vi "Interface.vi"() -> ()   [LabVIEW 2019, in "Command Interface.lvclass"]
uses:
  Command Interface.lvclass
  Robot/Universal Robot/Universal Robot.lvclass
  C:/_Code/Development/Sub-Zero Functional Test/standard hardware/Universal Robots/UR LabVIEW Interface/Classes/Application/Application Interfaces/Application Interface/Application Interface.lvclass
  Application.lvclass
  Application Interface/Application Interface.lvclass
panel:
  in  "Command":u16(ring) items=["Load", "Play", "Stop", "Pause", "Quit", "Shutdown", "Running", "Robotmode", "get loaded program", "popup", "close popup", "addToLog", "IsProgramSaved", "programState", "PolyscopeVersion", "set operational mode", "clear operational mode", "power on", "power off", "brake release", "safetystatus", "unlock protective stop", "close safety popup", "load installation", "restart safety", "get operational mode", "is in remote control", "get serial number", "get robot model", "generate flight report", "generate support file"]
  in  "Input":string
  out "Input Type":string
  in  "send":bool
  out "Return Status":string
  out "Data":string
  out "warning":string
  in  "interface":refnum<class "Command Interface.lvclass">
  in  "robot":refnum<class "Universal Robot.lvclass">
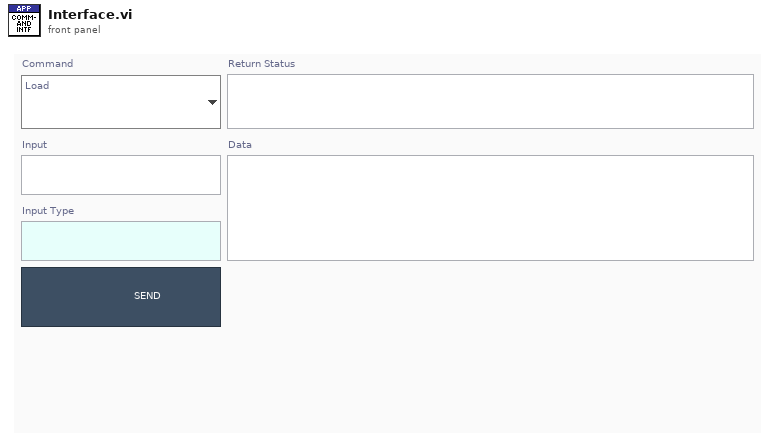
[diagram p1: front panel]
types:
  T1 = enum8{"Enabled", "Disabled", "Disabled and Grayed Out"}
  T2 = typedef "Application.lvclass/FrontPanelControls.ctl" = cluster{"Operation Interface":refnum<vi>, "Program Interface":refnum<vi>, "Command Interface":refnum<vi>, "Socket Interface":refnum<vi>, "Error Interface":refnum<vi>}
  T3 = typedef "Universal Robot.lvclass/PolyScopeCommand.ctl" = cluster{"Command":string, "Input":bool, "Input Type":string, "Remote Mode Required":bool, "Min Version":T4, "Deprecated":bool}
  T4 = typedef "Universal Robot.lvclass/PolyScopeVersion.ctl" = cluster{"Major":i32, "Minor":i32, "Fix":i32, "Build":i32}
  T5 = typedef "Universal Robot.lvclass/RobotStatus.ctl" = cluster{"Robot Mode":T6, "Operational Mode":T7, "Safety Status":T8, "Remote Control":bool}
  T6 = typedef "Universal Robot.lvclass/RobotMode.ctl" = enum16{"INVALID", "NO_CONTROLLER", "DISCONNECTED", "CONFIRM_SAFETY", "BOOTING", "POWER_OFF", "POWER_ON", "IDLE", "BACKDRIVE", "RUNNING"}
  T7 = typedef "Universal Robot.lvclass/OperationalMode.ctl" = enum16{"NONE", "MANUAL", "AUTOMATIC"}
  T8 = typedef "Universal Robot.lvclass/SafetyStatus.ctl" = enum16{"INVALID", "NORMAL", "REDUCED", "PROTECTIVE_STOP", "RECOVERY", "SAFEGUARD_STOP", "SYSTEM_EMERGENCY_STOP", "ROBOT_EMERGENCY_STOP", "VIOLATION", "FAULT", "AUTOMATIC_MODE_SAFEGAURD_STOP", "SYSTEM_THREE_POSITION_ENABLING_STOP"}
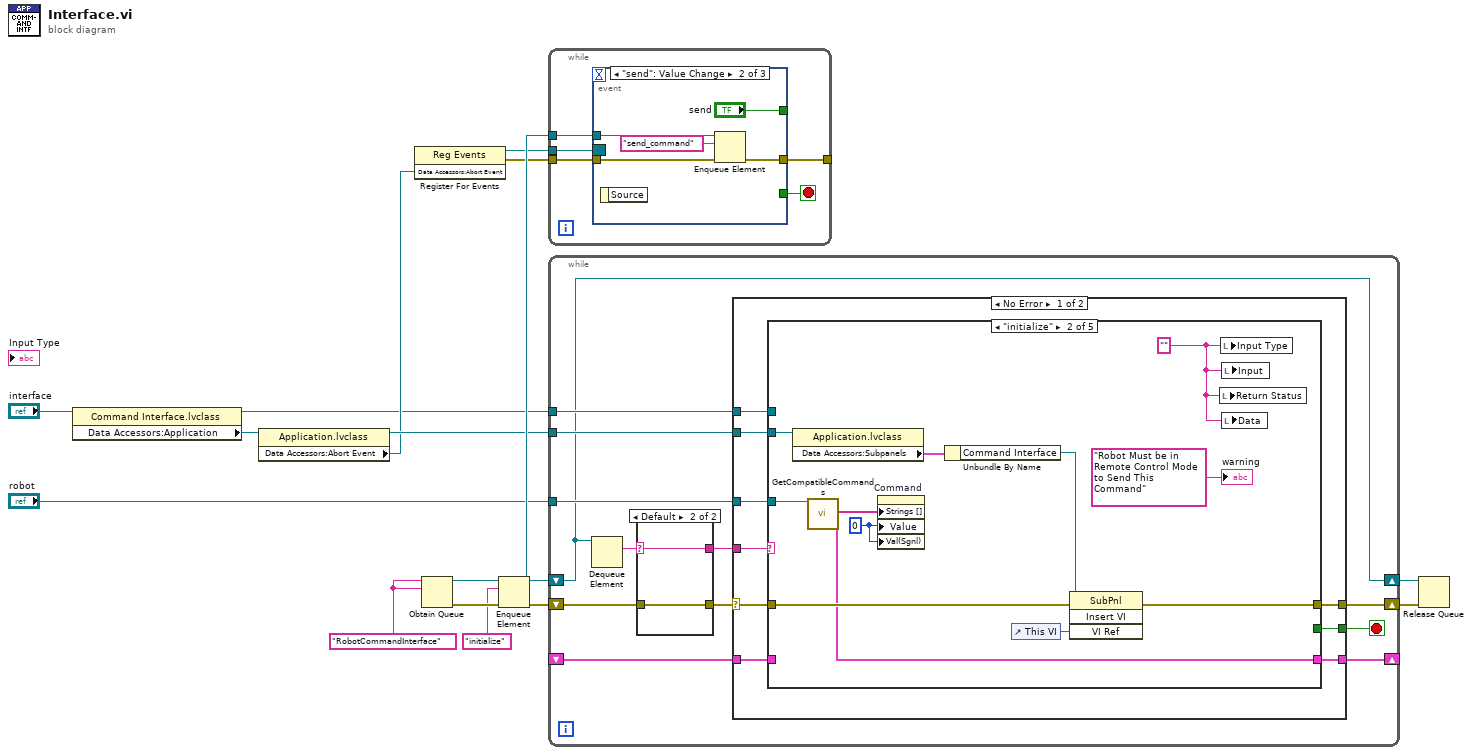
[diagram p0: block diagram]
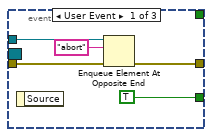
[diagram p2: hidden frame]
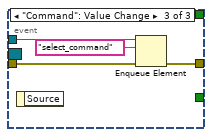
[diagram p3: hidden frame]
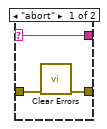
[diagram p4: hidden frame]
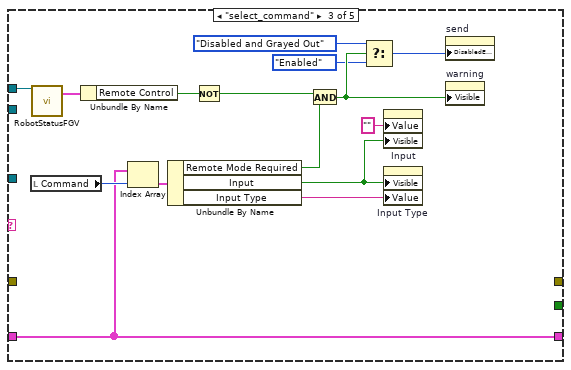
[diagram p6: hidden frame]
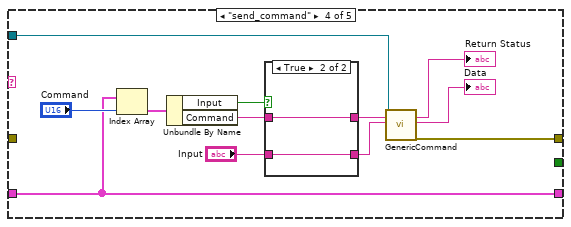
[diagram p7: hidden frame]
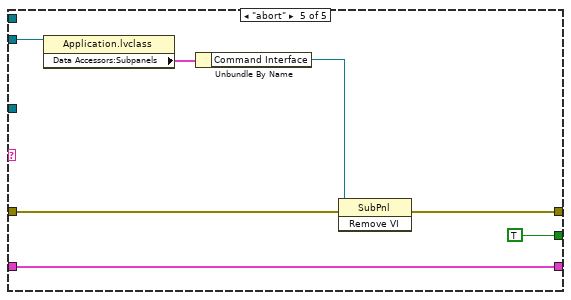
[diagram p9: hidden frame]
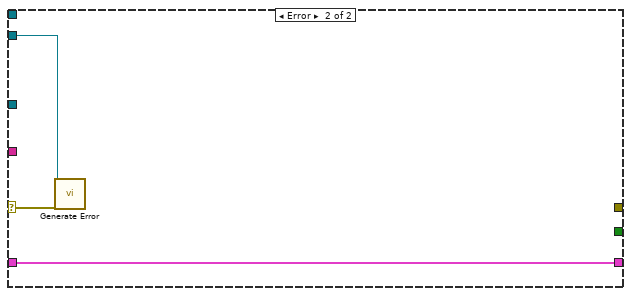
[diagram p10: hidden frame]
diagram:
  w11 = "RobotCommandInterface" ("name (unnamed)")
  n1 = property class="Command Interface.lvclass"(reference="interface") -> (reference out=w1:refnum<class "Command Interface.lvclass">, "Data Accessors:Application"=w5:refnum<class "Application.lvclass">)  [unwired: 1 in, 1 out]
  n2 = property class="Application.lvclass"(reference=w5) -> (reference out=w4:refnum<class "Application.lvclass">, "Data Accessors:Abort Event"=w3:refnum<user-event>)  [unwired: 1 in, 1 out]
  n3 = register-events(w3) -> (reference out=w7:refnum<event-registration>, error out=w8:errorcluster)  [unwired: 2 in]
  n4 = Obtain Queue(name (unnamed)=w11, element data type=w11) -> (queue out=w15:refnum<queue>, error out=w16:errorcluster)  [unwired: 3 in, 1 out]
  n5 = Enqueue Element(queue=w15, element="initialize", error in (no error)=w16) -> (queue out=w12:refnum<queue>, error out=w13:errorcluster)  [unwired: 1 in, 1 out]
  n6 = while {
    tunnel: w12 -> [w21]
    tunnel: w8 -> [w20]
    tunnel: w7 -> [w19]
    tunnel: [w18] -> _
    stop <- w17 stop-if-true
    n7 = event shown="[1] \"send\": Value Change" {
      selector: w19 -> [_ _ _]
      dyn-events: _ -> [_ _ _]
      timeout: _ -> [_ _ _]
      tunnel: w21 -> [w26 w31 w35]
      tunnel: w20 -> [w25 w30 w34]
      tunnel: [w24 w29 w33] -> w18
      tunnel: [TRUE _ _] -> w17
      tunnel: [_ "send" _] -> _
      event User Event {
        n8 = event-data() -> ()  [unwired: 1 in, 1 out]
        n9 = Enqueue Element At Opposite End(queue=w26, element="abort", error in (no error)=w25) -> (error out=w24:errorcluster)  [unwired: 1 in, 2 out]
      }
      event "send": Value Change {
        n10 = event-data() -> ()  [unwired: 1 in, 1 out]
        n11 = Enqueue Element(queue=w31, element="send_command", error in (no error)=w30) -> (error out=w29:errorcluster)  [unwired: 1 in, 2 out]
      }
      event "Command": Value Change {
        n12 = event-data() -> ()  [unwired: 1 in, 1 out]
        n13 = Enqueue Element(queue=w35, element="select_command", error in (no error)=w34) -> (error out=w33:errorcluster)  [unwired: 1 in, 2 out]
      }
    }
  }
  n14 = while {
    shift-right: [w47] -> w9
    shift-left: w13 -> [w40]
    shift-right: [w36] -> w10
    shift-left: w12 -> [w36]
    tunnel: w4 -> [w45]
    tunnel: "robot" -> [w44]
    shift-right: [w43] -> _
    shift-left: _ -> [w42]
    tunnel: w1 -> [w41]
    stop <- w46 stop-if-true
    n15 = Dequeue Element(queue=w36) -> (element=w38:string)  [unwired: 2 in, 3 out]
    n16 = case shown="Default" w38 {
      selector: w38 -> [w50 w51]
      tunnel: w40 -> [w48 w52]
      tunnel: [w49 w52] -> w39
      tunnel: [w50 w51] -> w37
      frame "abort" {
        n17 = call <vilib>:"Clear Errors.vi"("error in (no error)"=w48) -> ("error out"=w49:errorcluster)  [unwired: 5 in, 1 out]
      }
      frame Default {
      }
    }
    n18 = case shown="No Error" w39 {
      selector: w39 -> [w53 w113]
      tunnel: [w61 _] -> w47
      tunnel: [w60 _] -> w46
      tunnel: w45 -> [w59 w114]
      tunnel: w44 -> [w58 _]
      tunnel: [w57 w115] -> w43
      tunnel: w42 -> [w56 w115]
      tunnel: w41 -> [w55 _]
      tunnel: w37 -> [w54 _]
      frame No Error {
        n19 = case shown="\"initialize\"" w54 {
          tunnel: w53 -> [w63 w73 _ _ w106]
          tunnel: [w63 w75 _ w96 w111] -> w61
          tunnel: [_ _ _ _ TRUE] -> w60
          tunnel: w59 -> [_ w68 _ _ w109]
          tunnel: w58 -> [_ w71 _ w93 _]
          tunnel: [w62 w69 w89 w101 w110] -> w57
          tunnel: w56 -> [w62 _ w89 w101 w110]
          tunnel: w55 -> [_ _ w84 _ _]
          frame Default {
          }
          frame "initialize" {
            w64 = 0
            w72 = "" ("inputType")
            n20 = property class="Application.lvclass"(reference=w68) -> ("Data Accessors:Subpanels"=w67:T2)  [unwired: 1 in, 2 out]
            n21 = call-dynamic "GetCompatibleCommands.vi"("Universal Robot in"=w71) -> ("compatibleCommandList"=w70:string[], "compatibleCommands"=w69:T3[])  [unwired: 16 in, 1 out]
            n22 = property on="Command" class="Ring (strict)"("Strings []"=w70, "Value"=w64, "Val(Sgnl)"=w64) -> ()  [unwired: 2 in, 2 out]
            n23 = Unbundle By Name(w67) -> ("Command Interface"=w66:refnum<vi>)
            n24 = control-ref of="This VI"() -> (w74:refnum<vi>)
            n25 = invoke class="SubPnl" method="Insert VI"(reference=w66, error in=w73, "VI Ref"=w74) -> (error out=w75:errorcluster)  [unwired: 1 in, 3 out]
            n26 = local write "Return Status"(w72) -> ()
            n27 = local write "Input Type"(w72) -> ()
            n28 = local write "Input"(w72) -> ()
            n29 = local write "Data"(w72) -> ()
            "warning" <- "Robot Must be in Remote Control Mode to Send This Command" ("warning")
          }
          frame "select_command" {
            n30 = local read "Command"() -> (w90:u16)
            n31 = call "RobotStatusFGV.vi"("Application Interface in"=w84) -> ("Robot Status out"=w83:T5)  [unwired: 16 in, 2 out]
            n32 = Unbundle By Name(w83) -> ("Remote Control"=w81:bool)
            n33 = Index Array(array=w89, index=w90) -> (element=w88:T3)
            n34 = Unbundle By Name(w88) -> ("Remote Mode Required"=w82:bool, "Input"=w86:bool, "Input Type"=w87:string)
            n35 = Not(x=w81) -> (.not. x?=w80:bool)
            n36 = And(x=w80, y=w82) -> (x .and. y?=w79:bool)
            n37 = Select(t=T1."Disabled and Grayed Out" ("Disabled"), s=w79, f=T1."Enabled" ("Disabled")) -> (s? t:f=w76:T1)
            n38 = property on="Input" class="Str"("Value"="" ("input"), "Visible"=w86) -> ()  [unwired: 2 in, 2 out]
            n39 = property on="Input Type" class="Str"("Visible"=w86, "Value"=w87) -> ()  [unwired: 2 in, 2 out]
            n40 = property on="send" class="Bool"("DisabledEnum"=w76) -> ()  [unwired: 2 in, 2 out]
            n41 = property on="warning" class="Str"("Visible"=w79) -> ()  [unwired: 2 in, 2 out]
          }
          frame "send_command" {
            n42 = Index Array(array=w101, index="Command") -> (element=w100:T3)
            n43 = Unbundle By Name(w100) -> ("Input"=w99:bool, "Command"=w98:string)
            n44 = case shown="True" w99 {
              tunnel: w98 -> [w103 w105]
              tunnel: [w103 w105] -> w92
              tunnel: "Input" -> [_ w104]
              tunnel: [_ w104] -> w91
              frame False {
              }
              frame True {
              }
            }
            n45 = call-dynamic "GenericCommand.vi"("Universal Robot.lvclass in"=w93, "command"=w92, "data"=w91) -> ("returnStatus"=→"Return Status":string, "data out"=→"Data":string, "error out"=w96:errorcluster)  [unwired: 13 in, 1 out]
          }
          frame "abort" {
            n46 = property class="Application.lvclass"(reference=w109) -> ("Data Accessors:Subpanels"=w108:T2)  [unwired: 1 in, 2 out]
            n47 = Unbundle By Name(w108) -> ("Command Interface"=w107:refnum<vi>)
            n48 = invoke class="SubPnl" method="Remove VI"(reference=w107, error in=w106) -> (error out=w111:errorcluster)  [unwired: 1 in, 2 out]
          }
        }
      }
      frame Error {
        n49 = call "Generate Error.vi"("Application in"=w114, "error in (no error)"=w113) -> ()  [unwired: 17 in, 1 out]
      }
    }
  }
  n50 = Release Queue(queue=w10, error in (no error)=w9) -> ()  [unwired: 1 in, 3 out]
